vi "配置MES.vi"() -> (2 "MESPath":path, 3 "MES":T2)   [LabVIEW 2011]
uses:
  Button.ctl
  <vilib>/Utility/error.llb/DialogType.ctl
panel:
  in  "保存 2":T1
  in  "启用MES":bool
  in  "MES Config":T3
  in  "保存":T1
  out "Error Report":string
  in  "Temp":T4
  out "Error Out":errorcluster
  in  "Exit":T1
  # "MES配置"
  # "启用MES"
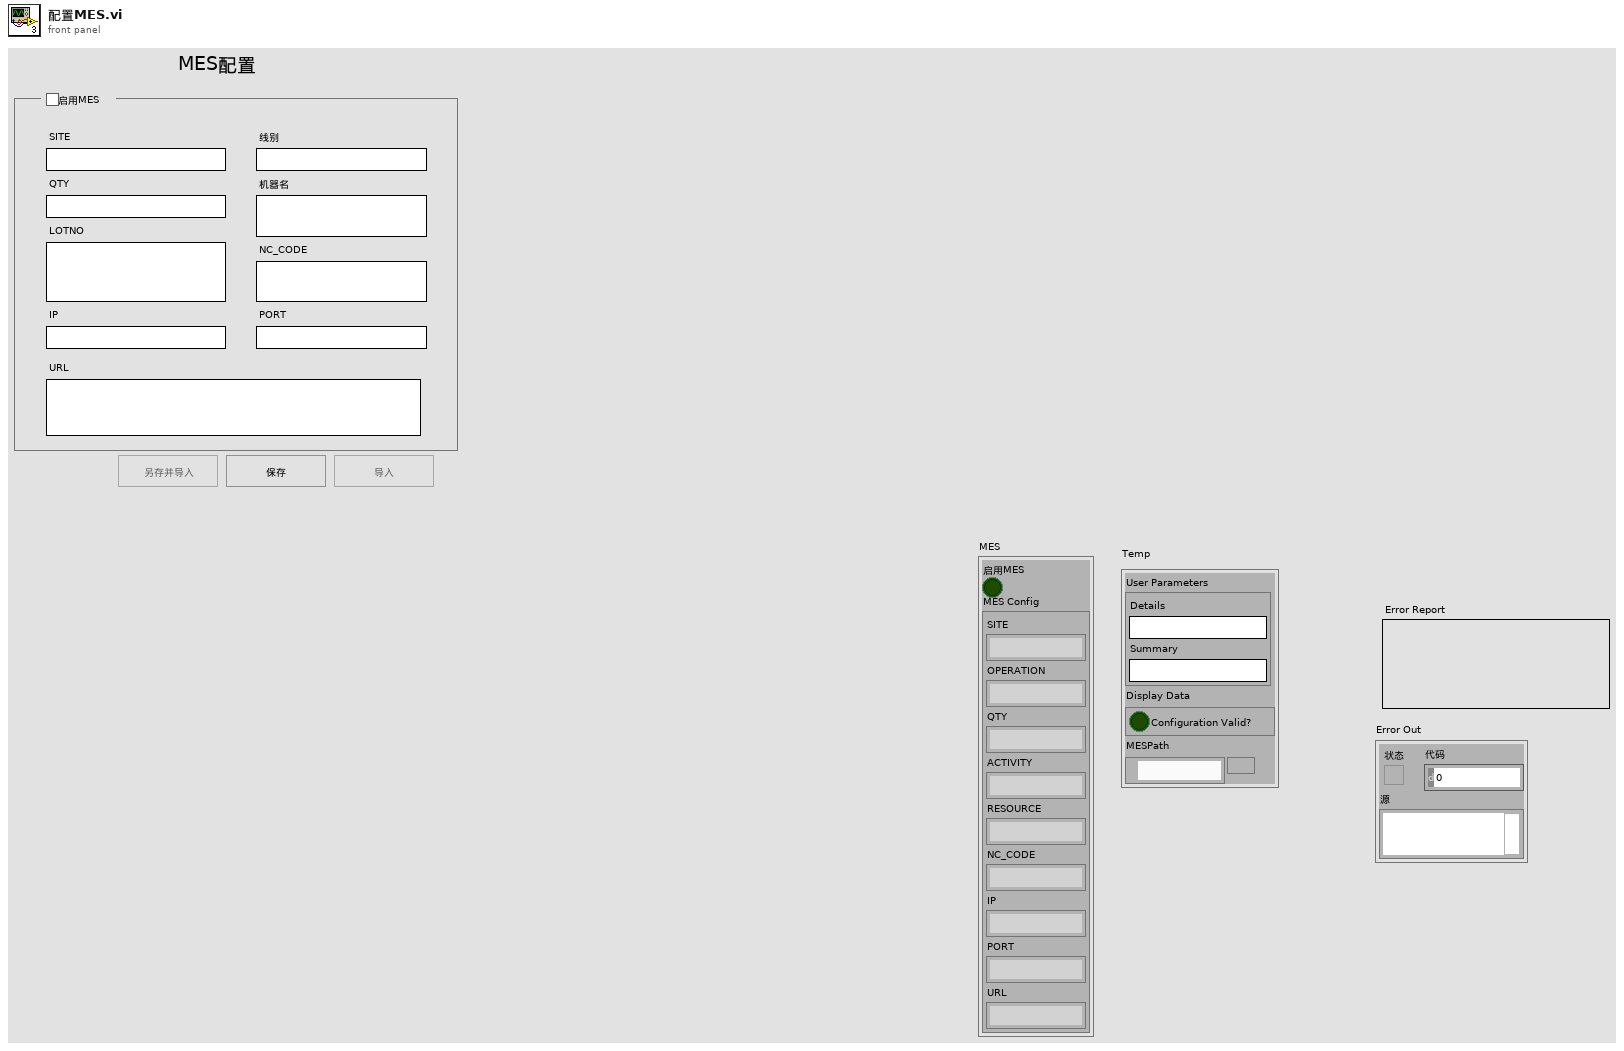
[diagram p1: front panel]
types:
  T1 = typedef "Button.ctl" = bool
  T2 = cluster{"启用MES":bool, "MES Config":cluster{"SITE":string, "OPERATION":string, "QTY":string, "ACTIVITY":string, "RESOURCE":string, "NC_CODE":string, "IP":string, "PORT":string, "URL":string}}
  T3 = cluster{"SITE":string, "线别":string, "QTY":string, "机器名":string, "LOTNO":string, "NC_CODE":string, "IP":string, "PORT":string, "URL":string}
  T4 = cluster{"User Parameters":cluster{"Details":string, "Summary":string}, "Display Data":cluster{"Configuration Valid?":bool}, "MESPath":path}
  T5 = cluster{"启用MES":bool, "MES Config":cluster{"SITE":string, "OPERATION":string, "QTY":string, "ACTIVITY":string, "RESOURCE":string, "NC_CODE":string, "IP":string, "PORT":string, "URL":string, "SFC":string}}
  T6 = cluster{"SITE":string, "OPERATION":string, "QTY":string, "ACTIVITY":string, "RESOURCE":string, "NC_CODE":string, "IP":string, "PORT":string, "URL":string, "SFC":string}
  T7 = enum32{"invalid app kind", "Development System", "Run Time System", "Student Edition", "Embedded LabVIEW", "Evaluation", "Custom"}
  T8 = typedef "amc_Message Queue.ctl" = refnum<queue>
  T9 = enum8{"Enabled", "Disabled", "Disabled and Grayed Out"}
  T10 = typedef "DialogType.ctl" = u16
  T11 = cluster{"SITE":string, "OPERATION":string, "QTY":string, "ACTIVITY":string, "RESOURCE":string, "NC_CODE":string, "IP":string, "PORT":string, "URL":string}
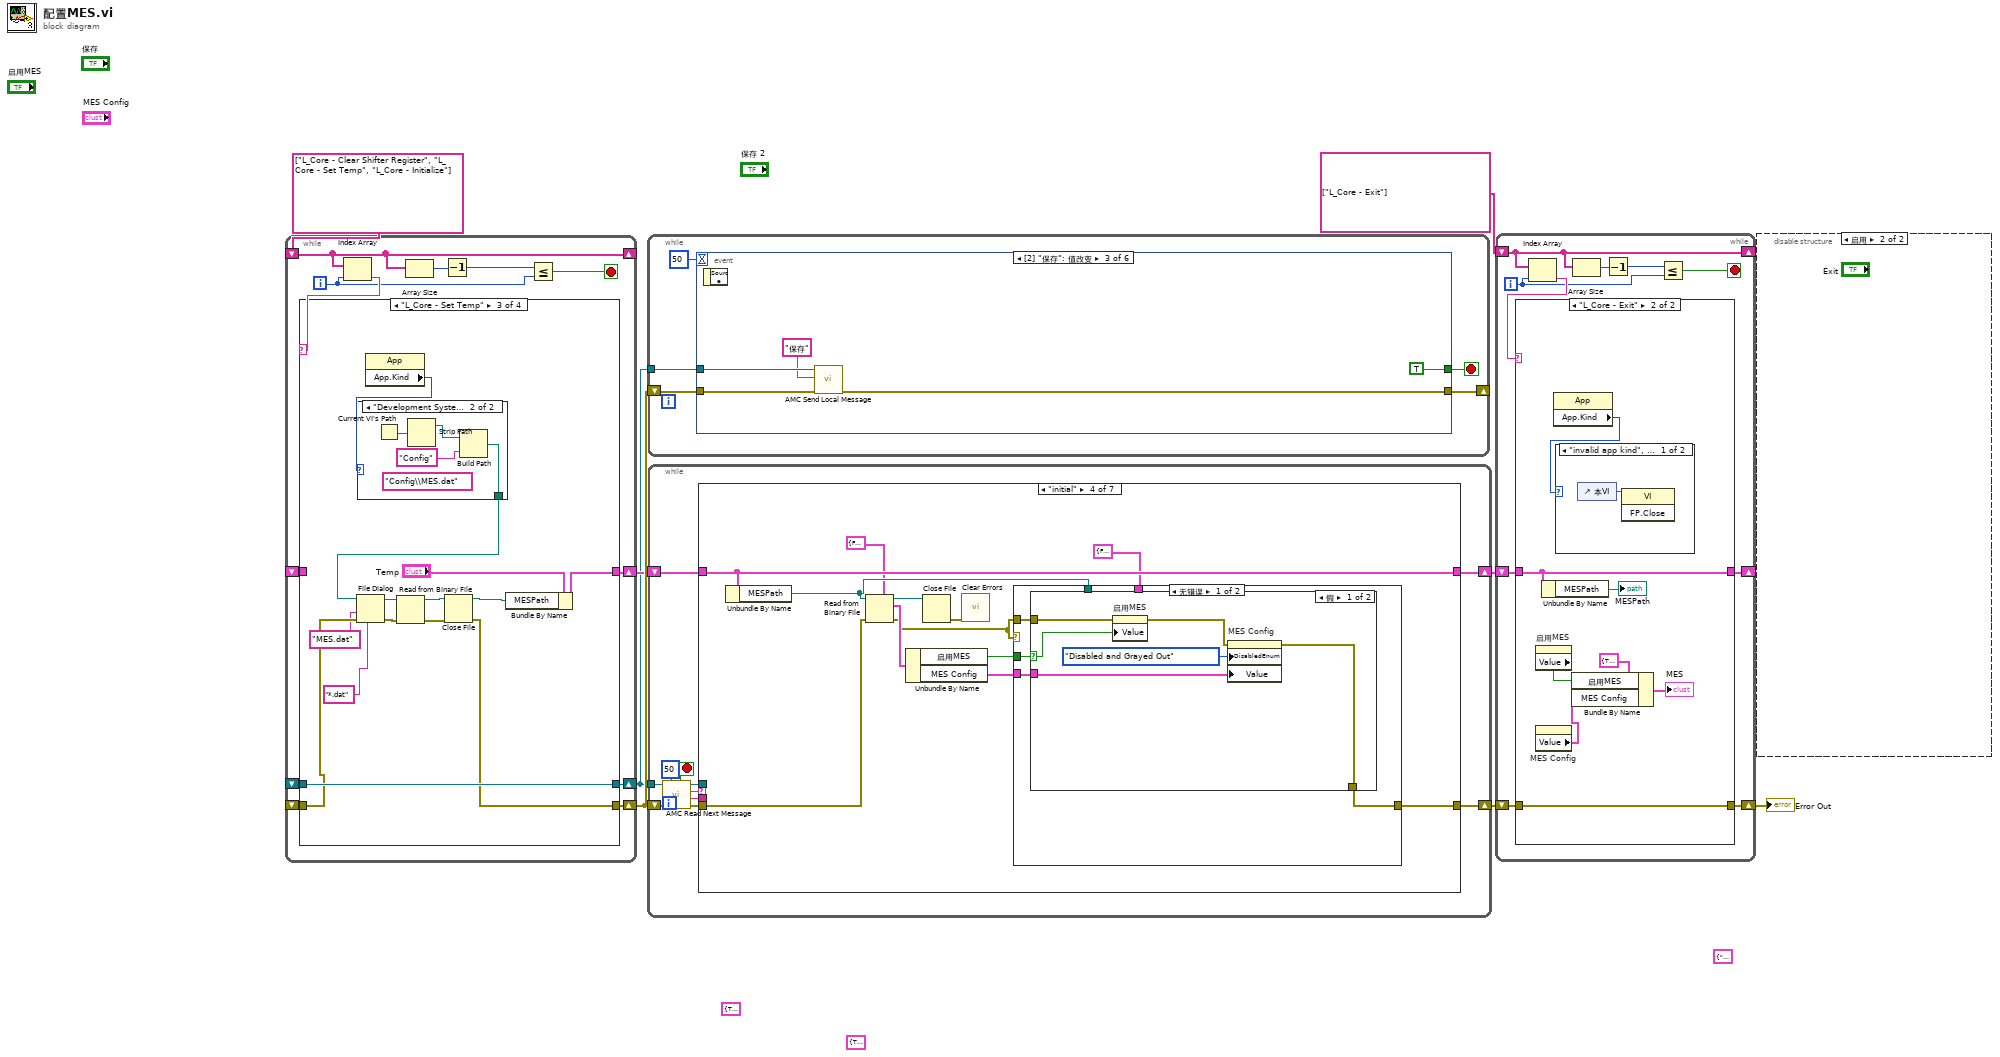
[diagram p0: block diagram]
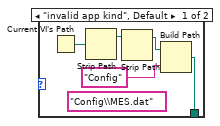
[diagram p7: hidden frame]
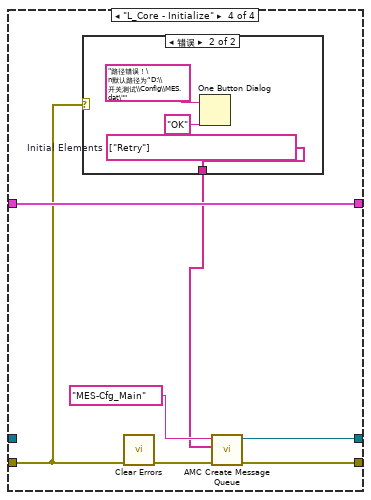
[diagram p8: hidden frame]
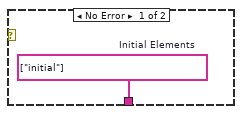
[diagram p9: hidden frame]
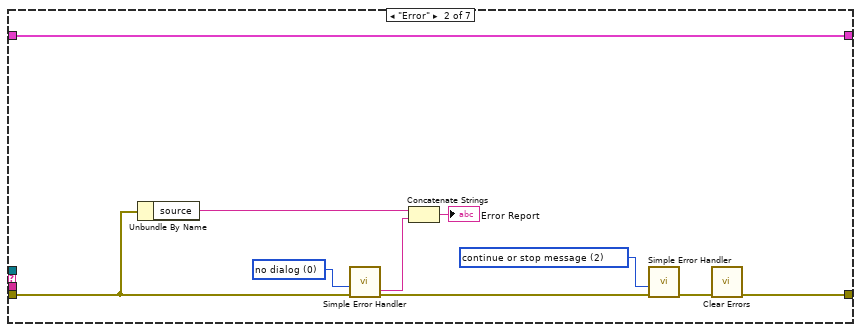
[diagram p11: hidden frame]
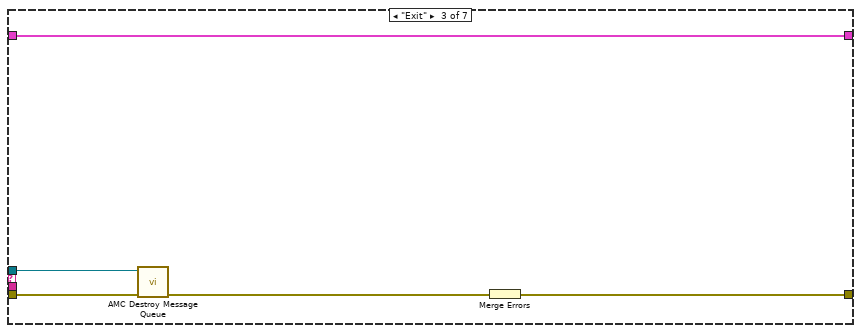
[diagram p12: hidden frame]
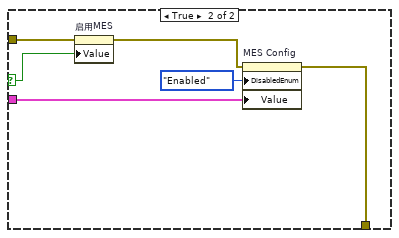
[diagram p13: hidden frame]
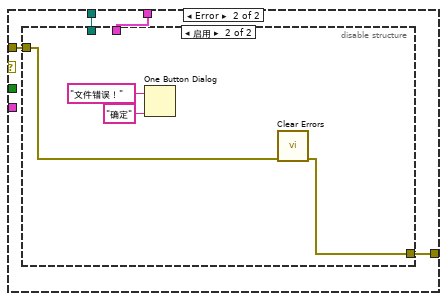
[diagram p14: hidden frame]
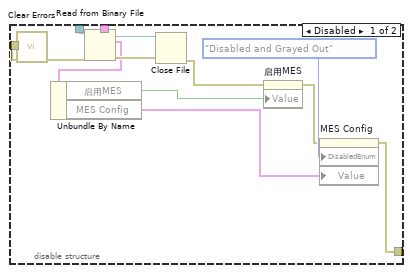
[diagram p15: hidden frame]
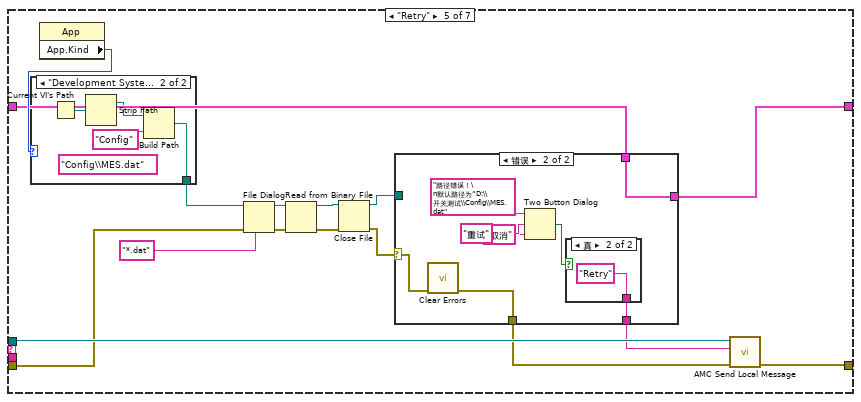
[diagram p16: hidden frame]
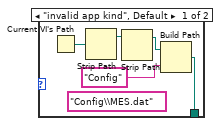
[diagram p17: hidden frame]
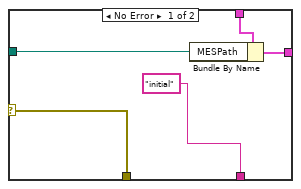
[diagram p18: hidden frame]
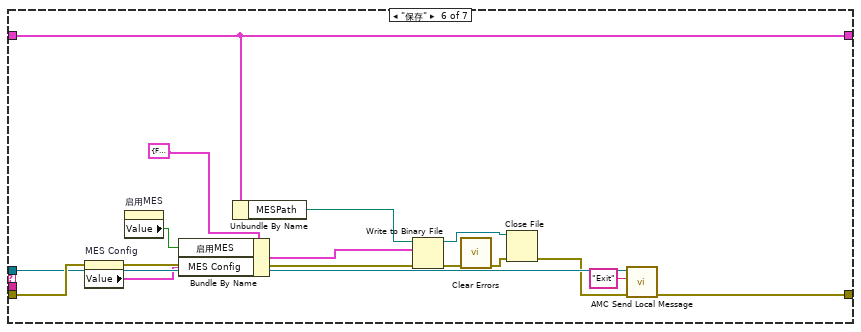
[diagram p20: hidden frame]
diagram:
  (unwired) T5 {"启用MES"=TRUE, "MES Config"={"SITE"="", "OPERATION"="", "QTY"="", "ACTIVITY"="", "RESOURCE"="", "NC_CODE"="", "IP"="", "PORT"="", "URL"="1\n1", "SFC"=""}}
  (unwired) T5 {"启用MES"=TRUE, "MES Config"={"SITE"="", "OPERATION"="", "QTY"="", "ACTIVITY"="", "RESOURCE"="", "NC_CODE"="", "IP"="", "PORT"="", "URL"="1\n1", "SFC"=""}}
  (unwired) T6 {"SITE"="", "OPERATION"="", "QTY"="", "ACTIVITY"="", "RESOURCE"="", "NC_CODE"="", "IP"="", "PORT"="", "URL"="1\n1", "SFC"=""} ("MES Config")
  n1 = while "App INIT" {
    shift-right: [w11] -> _
    shift-left: string[] ["L_Core - Clear Shifter Register", "L_Core - Set Temp", "L_Core - Initialize"] -> [w11]
    shift-right: [w20] -> w2
    shift-left: _ -> [w18]
    shift-right: [w19] -> w3
    shift-left: _ -> [w17]
    shift-right: [w10] -> w8
    shift-left: _ -> [w9]
    i -> [w15]
    stop <- w12 stop-if-true
    n2 = Index Array(array=w11, index=w15) -> (element=w16:string)
    n3 = case shown="\"L_Core - Set Temp\"" w16 {
      tunnel: [_ w24 w38 w53] -> w20
      tunnel: [w22 _ w35 w54] -> w19
      tunnel: w18 -> [_ w24 w38 _]
      tunnel: w17 -> [w22 _ _ w54]
      tunnel: [w21 w23 w31 w51] -> w10
      tunnel: w9 -> [w21 w23 w26 w50]
      frame "No Action", Default {
      }
      frame "L_Core - Clear Shifter Register" {
      }
      frame "L_Core - Set Temp" {
        n4 = property class="App"() -> ("App.Kind"=w37:T7)  [unwired: 2 in, 2 out]
        n5 = case shown="\"Development System\"" w37 {
          tunnel: [w40 w45] -> w28
          frame "invalid app kind", Default {
            (unwired) "Config\\MES.dat" ("名称或相对路径")
            n6 = Current VI's Path() -> (path=w43:path)
            n7 = Strip Path(path=w43) -> (stripped path=w42:path)  [unwired: 1 out]
            n8 = Strip Path(path=w42) -> (stripped path=w41:path)  [unwired: 1 out]
            n9 = Build Path(base path=w41, name or relative path="Config" ("名称或相对路径")) -> (appended path=w40:path)
          }
          frame "Development System" {
            (unwired) "Config\\MES.dat" ("名称或相对路径")
            n10 = Current VI's Path() -> (path=w47:path)
            n11 = Strip Path(path=w47) -> (stripped path=w46:path)  [unwired: 1 out]
            n12 = Build Path(base path=w46, name or relative path="Config" ("名称或相对路径")) -> (appended path=w45:path)
          }
        }
        n13 = File Dialog(6:"*.dat" ("数据类型"), 8:w26, 9:"MES.dat" ("默认名称"), 11:w28) -> (0:w27:errorcluster, 3:w30:path)  [unwired: 1 in, 4 out]
        n14 = Read from Binary File(8:w27, 11:w30) -> (0:w32:errorcluster, 3:w33:refnum<file>)  [unwired: 4 in, 2 out]
        n15 = Close File(refnum=w33, error in=w32) -> (path=w34:path, error out=w31:errorcluster)
        n16 = Bundle By Name(cluster="Temp", "MESPath"=w34) -> (w35:T4)
      }
      frame "L_Core - Initialize" {
        n17 = case shown="错误" w50 {
          tunnel: [w55 w56] -> w49
          frame No Error {
            w55 = string[] ["initial"]  # Initial Elements
          }
          frame Error {
            w56 = string[] ["Retry"]  # Initial Elements
            n18 = One Button Dialog(message="路径错误！\n默认路径为“D:\\开关测试\\Config\\MES.dat\"" ("消息"), button name ("OK")="OK" ("按钮名称（“确定”）")) -> ()  [unwired: 1 out]
          }
        }
        n19 = call <vilib>:"Clear Errors.vi"("error in (no error)"=w50) -> ("error out"=w48:errorcluster)  [unwired: 6 in]
        n20 = call <userlib>:"AMC Create Message Queue.vi"("error in (no error)"=w48, "Initial Message Names"=w49, "Message Queue Name"="MES-Cfg_Main") -> ("error out"=w51:errorcluster, "Message Queue out"=w53:T8)  [unwired: 7 in]
      }
    }
    n21 = Array Size(array=w11) -> (size(s)=w14:i32)
    n22 = Decrement(x=w14) -> (x-1=w13:i32)
    n23 = Less Or Equal?(x=w13, y=w15) -> (x <= y?=w12:bool)
  }
  n24 = while "Event Handler Loop" {
    tunnel: w2 -> [w62]
    shift-right: [w59] -> _
    shift-left: w8 -> [w60]
    stop <- w63 stop-if-true
    n25 = event shown="[2] \"保存\": 值改变" {
      selector: _ -> [_ _ _ _ _ _]
      dyn-events: _ -> [_ _ _ _ _ _]
      timeout: 50 -> [_ _ _ _ _ _]
      tunnel: [w65 TRUE ("NewVal") TRUE ("NewVal") TRUE ("NewVal") _ w90] -> w63
      tunnel: w62 -> [w66 w71 w76 w81 _ w88]
      tunnel: w60 -> [w64 w68 w73 w78 w83 w87]
      tunnel: [w64 w67 w72 w77 w83 w86] -> w59
      event Timeout {
        n26 = event-data() -> ()  [unwired: 2 out]
        n27 = Not A Number/Path/Refnum?(number/path/refnum=w66) -> (NaN/Path/Refnum?=w65:bool)
      }
      event Value Change {
        n28 = event-data() -> ()  [unwired: 2 out]
        n29 = call <userlib>:"AMC Send Local Message.vi"("error in (no error)"=w68, "Message Name"="Exit", "Message Queue in"=w71) -> ("error out"=w67:errorcluster)  [unwired: 7 in, 1 out]
      }
      event Value Change {
        n30 = event-data() -> ()  [unwired: 2 out]
        n31 = call <userlib>:"AMC Send Local Message.vi"("error in (no error)"=w73, "Message Name"="保存", "Message Queue in"=w76) -> ("error out"=w72:errorcluster)  [unwired: 7 in, 1 out]
      }
      event Value Change {
        n32 = event-data() -> ()  [unwired: 2 out]
        n33 = call <userlib>:"AMC Send Local Message.vi"("error in (no error)"=w78, "Message Name"="另存为", "Message Queue in"=w81) -> ("error out"=w77:errorcluster)  [unwired: 7 in, 1 out]
      }
      event "启用MES": Value Change {
        n34 = event-data() -> ("NewVal"=w82:bool)  [unwired: 1 out]
        n35 = case shown="真" w82 {
          frame False {
            n36 = property on="MES Config" class="Clust (严格)"("DisabledEnum"=T9."Disabled and Grayed Out" ("禁用")) -> ()  [unwired: 2 in, 2 out]
          }
          frame True {
            n37 = property on="MES Config" class="Clust (严格)"("DisabledEnum"=T9."Enabled" ("禁用")) -> ()  [unwired: 2 in, 2 out]
          }
        }
      }
      event Panel Close? {
        w90 = TRUE  # Discard?
        n38 = event-data() -> ()  [unwired: 5 out]
        n39 = call <userlib>:"AMC Send Local Message.vi"("error in (no error)"=w87, "Message Name"="Exit", "Message Queue in"=w88) -> ("error out"=w86:errorcluster)  [unwired: 7 in, 1 out]
        n40 = event-data("Discard?"=w90) -> ()  [unwired: 1 in, 1 out]
      }
    }
  }
  n41 = while "Primary Execution Loop" {
    shift-right: [w94] -> w1
    shift-left: w3 -> [w95]
    tunnel: w2 -> [w101]
    shift-right: [w93] -> w6
    shift-left: w8 -> [w92]
    stop <- w98 stop-if-true
    n42 = call <userlib>:"AMC Read Next Message.vi"("error in (no error)"=w92, "timeout (1ms)"=50, "Message Queue in"=w101) -> ("error out"=w99:errorcluster, "Message Value"=w96:string, "Message Name"=w97:string, "Message Queue out"=w100:T8, "Exit Process"=w98:bool)  [unwired: 2 in, 2 out]
    n43 = case shown="\"initial\"" w97 {
      tunnel: [w102 w105 w117 w125 w178 w215 w231] -> w93
      tunnel: w99 -> [w102 w107 w116 w126 w173 w220 w235]
      tunnel: w100 -> [_ _ w115 _ w180 w217 w233]
      tunnel: w95 -> [w103 w113 w118 w130 w169 w219 w234]
      tunnel: [w103 w113 w118 w130 w168 w219 w234] -> w94
      tunnel: w96 -> [_ _ _ _ _ _ _]
      frame "No Action", Default {
      }
      frame "Error" {
        w109 = T10 0 items=["no dialog", "OK message", "continue or stop message", "OK message + warnings", "continue/stop + warnings"] ("type of dialog (OK msg:1)")
        w110 = T10 2 items=["no dialog", "OK message", "continue or stop message", "OK message + warnings", "continue/stop + warnings"] ("type of dialog (OK msg:1)")
        n44 = Unbundle By Name(w107) -> ("source"=w112:string)
        n45 = call <vilib>:"Simple Error Handler.vi"("type of dialog (OK msg:1)"=w109, "error in (no error)"=w107) -> ("error out"=w108:errorcluster, "message"=w106:string)  [unwired: 3 in, 3 out]
        n46 = Concatenate Strings(w112, w106) -> (→"Error Report":string)
        n47 = call <vilib>:"Simple Error Handler.vi"("type of dialog (OK msg:1)"=w110, "error in (no error)"=w108) -> ("error out"=w111:errorcluster)  [unwired: 3 in, 4 out]
        n48 = call <vilib>:"Clear Errors.vi"("error in (no error)"=w111) -> ("error out"=w105:errorcluster)  [unwired: 6 in]
      }
      frame "Exit" {
        n49 = call <userlib>:"AMC Destroy Message Queue.vi"("error in (no error)"=w116, "Message Queue in"=w115) -> ("error out"=w114:errorcluster)  [unwired: 8 in, 1 out]
        n50 = Merge Errors(w114) -> (w117:errorcluster)
      }
      frame "initial" {
        n51 = Unbundle By Name(w130) -> ("MESPath"=w124:path)
        n52 = Read from Binary File(5:T2 {"启用MES"=FALSE, "MES Config"={"SITE"="", "OPERATION"="", "QTY"="", "ACTIVITY"="", "RESOURCE"="", "NC_CODE"="", "IP"="", "PORT"="", "URL"=""}} ("MES 2"), 8:w126, 11:w124) -> (0:w122:errorcluster, 2:w129:T2, 3:w123:refnum<file>)  [unwired: 3 in, 1 out]
        n53 = Unbundle By Name(w129) -> ("启用MES"=w128:bool, "MES Config"=w127:T11)
        n54 = Close File(refnum=w123) -> (error out=w121:errorcluster)  [unwired: 1 in, 1 out]
        n55 = call <vilib>:"Clear Errors.vi"("error in (no error)"=w121) -> ()  [unwired: 6 in, 1 out]
        n56 = case shown="无错误" w122 {
          tunnel: w128 -> [w134 _]
          tunnel: w127 -> [w133 _]
          tunnel: w122 -> [w132 w150]
          tunnel: [w131 w147] -> w125
          tunnel: w124 -> [_ w149]
          tunnel: T2 {"启用MES"=FALSE, "MES Config"={"SITE"="", "OPERATION"="", "QTY"="", "ACTIVITY"="", "RESOURCE"="", "NC_CODE"="", "IP"="", "PORT"="", "URL"=""}} ("MES 2") -> [_ w148]
          frame No Error {
            n57 = case shown="假" w134 {
              selector: w134 -> [w138 w144]
              tunnel: w133 -> [w139 w145]
              tunnel: w132 -> [w136 w142]
              tunnel: [w135 w141] -> w131
              frame False {
                n58 = property on="启用MES" class="Bool (严格)"(error in=w136, "Value"=w138) -> (error out=w137:errorcluster)  [unwired: 1 in, 1 out]
                n59 = property on="MES Config" class="Clust (严格)"(error in=w137, "DisabledEnum"=T9."Disabled and Grayed Out" ("禁用"), "Value"=w139) -> (error out=w135:errorcluster)  [unwired: 1 in, 1 out]
              }
              frame True {
                n60 = property on="启用MES" class="Bool (严格)"(error in=w142, "Value"=w144) -> (error out=w143:errorcluster)  [unwired: 1 in, 1 out]
                n61 = property on="MES Config" class="Clust (严格)"(error in=w143, "DisabledEnum"=T9."Enabled" ("禁用"), "Value"=w145) -> (error out=w141:errorcluster)  [unwired: 1 in, 1 out]
              }
            }
          }
          frame Error {
            n62 = disable-structure shown="启用" {
              disable-tunnel: w150 -> [w163 w167]
              disable-tunnel: w149 -> [w162 _]
              disable-tunnel: w148 -> [w161 _]
              disable-tunnel: [w151 w166] -> w147
              frame Disabled {
                n63 = call <vilib>:"Clear Errors.vi"("error in (no error)"=w163) -> ("error out"=w160:errorcluster)  [unwired: 6 in]
                n64 = Read from Binary File(5:w161, 8:w160, 11:w162) -> (0:w158:errorcluster, 2:w153:T2, 3:w159:refnum<file>)  [unwired: 3 in, 1 out]
                n65 = Unbundle By Name(w153) -> ("启用MES"=w155:bool, "MES Config"=w152:T11)
                n66 = Close File(refnum=w159, error in=w158) -> (error out=w154:errorcluster)  [unwired: 1 out]
                n67 = property on="启用MES" class="Bool (严格)"(error in=w154, "Value"=w155) -> (error out=w156:errorcluster)  [unwired: 1 in, 1 out]
                n68 = property on="MES Config" class="Clust (严格)"(error in=w156, "DisabledEnum"=T9."Disabled and Grayed Out" ("禁用"), "Value"=w152) -> (error out=w151:errorcluster)  [unwired: 1 in, 1 out]
              }
              frame Enabled {
                n69 = One Button Dialog(message="文件错误！" ("消息"), button name ("OK")="确定" ("按钮名称（“确定”）")) -> ()  [unwired: 1 out]
                n70 = call <vilib>:"Clear Errors.vi"("error in (no error)"=w167) -> ("error out"=w166:errorcluster)  [unwired: 6 in]
              }
            }
          }
        }
      }
      frame "Retry" {
        n71 = property class="App"() -> ("App.Kind"=w172:T7)  [unwired: 2 in, 2 out]
        n72 = case shown="\"Development System\"" w172 {
          tunnel: [w185 w190] -> w171
          frame "invalid app kind", Default {
            (unwired) "Config\\MES.dat" ("名称或相对路径")
            n73 = Current VI's Path() -> (path=w188:path)
            n74 = Strip Path(path=w188) -> (stripped path=w187:path)  [unwired: 1 out]
            n75 = Strip Path(path=w187) -> (stripped path=w186:path)  [unwired: 1 out]
            n76 = Build Path(base path=w186, name or relative path="Config" ("名称或相对路径")) -> (appended path=w185:path)
          }
          frame "Development System" {
            (unwired) "Config\\MES.dat" ("名称或相对路径")
            n77 = Current VI's Path() -> (path=w192:path)
            n78 = Strip Path(path=w192) -> (stripped path=w191:path)  [unwired: 1 out]
            n79 = Build Path(base path=w191, name or relative path="Config" ("名称或相对路径")) -> (appended path=w190:path)
          }
        }
        n80 = File Dialog(6:"*.dat" ("数据类型"), 8:w173, 11:w171) -> (0:w174:errorcluster, 3:w175:path)  [unwired: 1 in, 5 out]
        n81 = Read from Binary File(8:w174, 11:w175) -> (0:w183:errorcluster, 3:w182:refnum<file>)  [unwired: 4 in, 2 out]
        n82 = Close File(refnum=w182, error in=w183) -> (path=w170:path, error out=w181:errorcluster)
        n83 = case shown="错误" w181 {
          selector: w181 -> [w196 w200]
          tunnel: ["initial" w204] -> w179
          tunnel: [w196 w199] -> w177
          tunnel: w169 -> [w195 w198]
          tunnel: w170 -> [w194 _]
          tunnel: [w193 w198] -> w168
          frame No Error {
            n84 = Bundle By Name(cluster=w195, "MESPath"=w194) -> (w193:T4)
          }
          frame Error {
            n85 = call <vilib>:"Clear Errors.vi"("error in (no error)"=w200) -> ("error out"=w199:errorcluster)  [unwired: 6 in]
            n86 = Two Button Dialog(message="路径错误！\n默认路径为“D:\\开关测试\\Config\\MES.dat" ("消息"), 1:"取消" ("F按钮名称（“取消”）"), 2:"重试" ("按钮名称（“确定”）")) -> (T button?=w201:bool)
            n87 = case shown="真" w201 {
              tunnel: [_ "Retry"] -> w204
              frame False {
              }
              frame True {
              }
            }
          }
        }
        n88 = call <userlib>:"AMC Send Local Message.vi"("error in (no error)"=w177, "Message Name"=w179, "Message Queue in"=w180) -> ("error out"=w178:errorcluster)  [unwired: 7 in, 1 out]
      }
      frame "保存" {
        n89 = property on="MES Config" class="Clust (严格)"(error in=w220) -> (error out=w221:errorcluster, "Value"=w213:T3)  [unwired: 1 in, 1 out]
        n90 = property on="启用MES" class="Bool (严格)"() -> ("Value"=w211:bool)  [unwired: 2 in, 2 out]
        n91 = Bundle By Name(cluster=T2 {"启用MES"=FALSE, "MES Config"={"SITE"="", "OPERATION"="", "QTY"="", "ACTIVITY"="", "RESOURCE"="", "NC_CODE"="", "IP"="", "PORT"="", "URL"=""}} ("MES 2"), "启用MES"=w211, "MES Config"=w213) -> (w212:T2)
        n92 = Unbundle By Name(w219) -> ("MESPath"=w218:path)
        n93 = Write to Binary File(file (use dialog)=w218, data=w212, error in=w221) -> (refnum out=w209:refnum<file>, error out=w216:errorcluster)  [unwired: 3 in, 1 out]
        n94 = call <vilib>:"Clear Errors.vi"("error in (no error)"=w216) -> ("error out"=w208:errorcluster)  [unwired: 6 in]
        n95 = Close File(refnum=w209, error in=w208) -> (error out=w210:errorcluster)  [unwired: 1 out]
        n96 = call <userlib>:"AMC Send Local Message.vi"("error in (no error)"=w210, "Message Name"="Exit", "Message Queue in"=w217) -> ("error out"=w215:errorcluster)  [unwired: 7 in, 1 out]
      }
      frame "另存为" {
        n97 = property on="MES Config" class="Clust (严格)"(error in=w235) -> (error out=w236:errorcluster, "Value"=w229:T3)  [unwired: 1 in, 1 out]
        n98 = property on="启用MES" class="Bool (严格)"() -> ("Value"=w227:bool)  [unwired: 2 in, 2 out]
        n99 = Bundle By Name(cluster=T2 {"启用MES"=FALSE, "MES Config"={"SITE"="", "OPERATION"="", "QTY"="", "ACTIVITY"="", "RESOURCE"="", "NC_CODE"="", "IP"="", "PORT"="", "URL"=""}} ("MES 2"), "启用MES"=w227, "MES Config"=w229) -> (w228:T2)
        n100 = Write to Binary File(data=w228, error in=w236, 7:"*.dat" ("提示（选择或输入文件路径）")) -> (refnum out=w225:refnum<file>, error out=w232:errorcluster)  [unwired: 3 in, 1 out]
        n101 = call <vilib>:"Clear Errors.vi"("error in (no error)"=w232) -> ("error out"=w224:errorcluster)  [unwired: 6 in]
        n102 = Close File(refnum=w225, error in=w224) -> (error out=w226:errorcluster)  [unwired: 1 out]
        n103 = call <userlib>:"AMC Send Local Message.vi"("error in (no error)"=w226, "Message Name"="Exit", "Message Queue in"=w233) -> ("error out"=w231:errorcluster)  [unwired: 7 in, 1 out]
      }
    }
  }
  n104 = while "App Close" {
    shift-right: [w239] -> _
    shift-left: string[] ["L_Core - Exit"] -> [w239]
    shift-right: [w245] -> _
    shift-left: w1 -> [w246]
    shift-right: [w237] -> w7
    shift-left: w6 -> [w238]
    i -> [w241]
    stop <- w240 stop-if-true
    n105 = Index Array(array=w239, index=w241) -> (element=w242:string)
    n106 = case shown="\"L_Core - Exit\"" w242 {
      tunnel: [w248 w250] -> w245
      tunnel: w246 -> [w248 w250]
      tunnel: w238 -> [w247 w256]
      tunnel: [w247 w256] -> w237
      frame "No Action", Default {
      }
      frame "L_Core - Exit" {
        n107 = property on="启用MES" class="Bool (严格)"() -> ("Value"=w254:bool)  [unwired: 2 in, 2 out]
        n108 = property on="MES Config" class="Clust (严格)"() -> ("Value"=w253:T3)  [unwired: 2 in, 2 out]
        n109 = Unbundle By Name(w250) -> ("MESPath"=→"MESPath":path)
        n110 = property class="App"() -> ("App.Kind"=w255:T7)  [unwired: 2 in, 2 out]
        n111 = case shown="\"invalid app kind\", 默认" w255 {
          frame "invalid app kind", Default {
            n112 = control-ref of="本VI"() -> (w257:refnum<vi>)
            n113 = invoke class="VI" method="FP.Close"(reference=w257) -> ()  [unwired: 2 in, 3 out]
          }
          frame "Development System" {
          }
        }
        n114 = Bundle By Name(cluster=T2 {"启用MES"=TRUE, "MES Config"={"SITE"="", "OPERATION"="", "QTY"="", "ACTIVITY"="", "RESOURCE"="", "NC_CODE"="", "IP"="", "PORT"="", "URL"="1\n1"}}, "启用MES"=w254, "MES Config"=w253) -> (→"MES":T2)
      }
    }
    n115 = Array Size(array=w239) -> (size(s)=w244:i32)
    n116 = Decrement(x=w244) -> (x-1=w243:i32)
    n117 = Less Or Equal?(x=w243, y=w241) -> (x <= y?=w240:bool)
  }
  "Error Out" <- w7
  n118 = disable-structure shown="启用" {
    frame Disabled {
    }
    frame Enabled {
    }
  }
